vi "solar_excel Workbook Get Sheets.vi"(8 "error in (no error)":errorcluster, 11 "Excel Workbook in":T1) -> (0 "error out":errorcluster, 1 "Worksheet Count":i32, 2 "Worksheet Names":string[](array[string]), 3 "Excel Workbook out":T1)   [LabVIEW 2018]
doc: "This returns a list of all Worksheets in the active Workbook reference."
uses:
  solar_excel_ctl Workbook.ctl
  solar_excel_ctl TSV.ctl
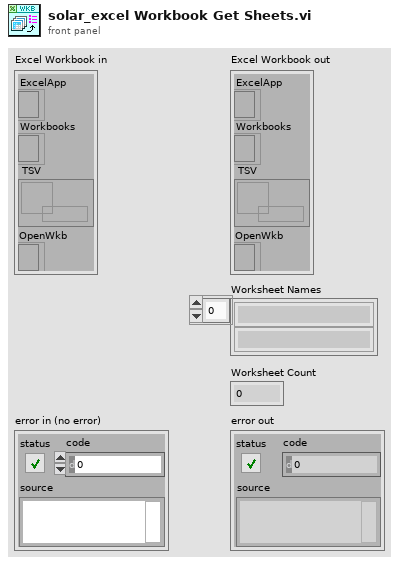
[diagram p1: front panel]
types:
  T1 = typedef "solar_excel_ctl Workbook.ctl" = cluster{"ExcelApp":refnum<k7>, "Workbooks":refnum<k7>, "TSV":refnum<queue>, "OpenWkb":refnum<k7>}
  T2 = typedef "solar_excel_ctl TSV.ctl" = cluster{"Path":path, "Dirty":bool, "ActiveSheet":u8, "Worksheets":string[], "Worksheet Cells":cluster{"Cells":string[][]}[]}
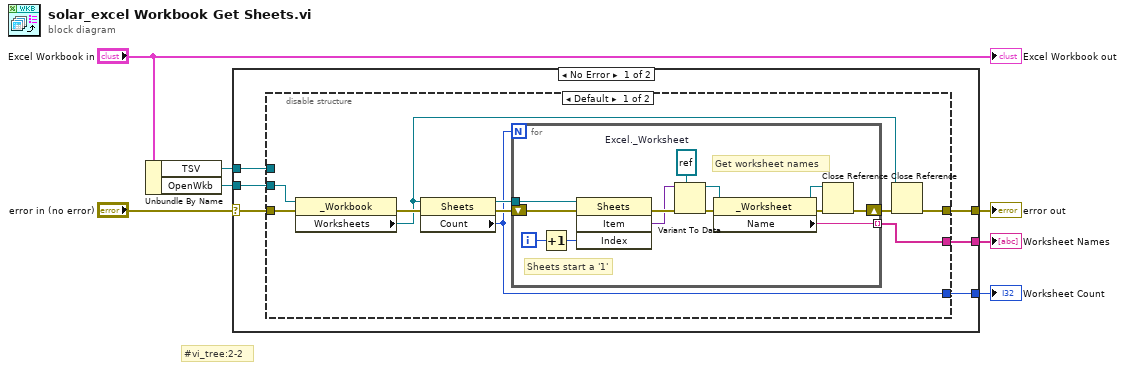
[diagram p0: block diagram]
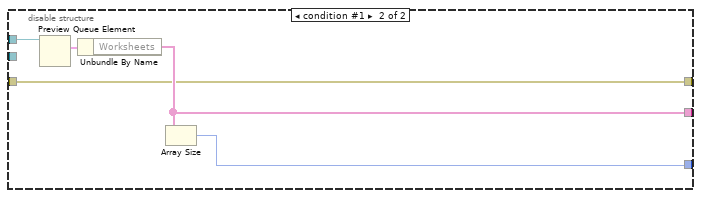
[diagram p2: hidden frame]
diagram:
  # "#vi_tree:2-2"
  n1 = Unbundle By Name("Excel Workbook in") -> ("TSV"=w1:refnum<queue>, "OpenWkb"=w5:refnum<k7>)
  n2 = case shown="No Error" "error in (no error)" {
    selector: "error in (no error)" -> [w13 w42]
    tunnel: [w11 w42] -> w7
    tunnel: w5 -> [w12 _]
    tunnel: [w10 _] -> w3
    tunnel: [w9 _] -> w2
    tunnel: w1 -> [w8 _]
    frame No Error {
      n3 = disable-structure shown="Default" {
        disable-tunnel: w13 -> [w23 w38]
        disable-tunnel: w12 -> [w21 _]
        disable-tunnel: [w17 w38] -> w11
        disable-tunnel: [w15 w37] -> w10
        disable-tunnel: [w14 w39] -> w9
        disable-tunnel: w8 -> [_ w41]
        frame condition #0 (active) {
          n4 = property class="_Workbook"(reference=w21, error in=w23) -> (error out=w22:errorcluster, "Worksheets"=w16:refnum<k7>)  [unwired: 1 out]
          n5 = property class="Sheets"(reference=w16, error in=w22) -> (reference out=w18:refnum<k7>, error out=w19:errorcluster, "Count"=w15:i32)
          n6 = for {
            N: w15 -> [_]
            shift-right: [w26] -> w20
            shift-left: w19 -> [w32]
            tunnel: w18 -> [w31]
            tunnel: [w24] -> w14 mode=indexing
            i -> [w30]
            w33 = refnum<k7> refnum  # Excel._Worksheet
            # "Get worksheet names"
            # "Sheets start a '1'"
            n7 = Increment(x=w30) -> (x+1=w29:i32)
            n8 = invoke class="Sheets" method="Item"(reference=w31, error in=w32, "Index"=w29) -> (error out=w36:errorcluster, "Item"=w34:variant)  [unwired: 1 in, 2 out]
            n9 = Variant To Data(error in=w36, type=w33, Variant=w34) -> (data=w27:refnum<k7>, error out=w35:errorcluster)
            n10 = property class="_Worksheet"(reference=w27, error in=w35) -> (reference out=w25:refnum<k7>, error out=w28:errorcluster, "Name"=w24:string)
            n11 = Close Reference(reference=w25, error in (no error)=w28) -> (error out=w26:errorcluster)
          }
          n12 = Close Reference(reference=w16, error in (no error)=w20) -> (error out=w17:errorcluster)
        }
        frame condition #1 {
          n13 = Preview Queue Element(queue=w41) -> (element=w40:T2)  [unwired: 2 in, 3 out]
          n14 = Unbundle By Name(w40) -> ("Worksheets"=w39:string[])
          n15 = Array Size(array=w39) -> (size(s)=w37:i32)
        }
      }
    }
    frame Error {
    }
  }
  "error out" <- w7
  "Worksheet Count" <- w3
  "Worksheet Names" <- w2
  "Excel Workbook out" <- "Excel Workbook in"
